vi "Tracker_v.2.2+.vi"() -> ()   [LabVIEW 2018]
uses:
  SubVi's/Controls/CTL_IO_parameters_indicator.ctl
  SubVi's/Controls/CTL_Zones_control_and_indicator.ctl
  SubVi's/Controls/CTL_All_References.ctl
  SubVi's/Controls/CTL_Controls_References.ctl
  SubVi's/Controls/CTL_Indicators_References.ctl
  SubVi's/Controls/CTL_Panes_and_VIs_References.ctl
  <vilib>/event_ctls.llb/eventsource.ctl
  SubVi's/Controls/CTL_Control_States.ctl
  <vilib>/Platform/TimedLoop/XDataNode/timing_clust.ctl
  <vilib>/Platform/TimedLoop/XDataNode/nitl_modes.ctl
  <vilib>/Platform/TimedLoop/XDataNode/wakeup.ctl
  <vilib>/Utility/error.llb/DialogType.ctl
  <vilib>/Instr/_visa.llb/VISA Flush IO Buffer Mask.ctl
  SubVi's/SW_Globals_2.2+.vi
  <vilib>/Platform/TimedLoop/scheduler/LVUserAPI/_suppVIs/Create_1kHz_TSource.vi
  <vilib>/platform/TimedLoop/XDataNode/XDataNode.xnode
  <vilib>/Platform/TimedLoop/XDataNode/XDNodeRunTimeDep.lvlib
panel:
  out "ItemPath":string
  out "ItemTag":string
  out "Source":T1 items=["LabVIEW UI"=0, "ActiveX"=1, "User Event"=25]
  out "Timing Source":string
  in  "Show magnets":bool=TRUE caption="Magnets"
  in  "Panes references":T2
  in  "Indicators references":T3
  in  "Controls references":T4
  in  "All references":T5
  out "Experiment Diagram":T6(plugin-control)
  in  "Reset barplot":bool
  out "Mouse speed, mm/s":dbl=0.28949046360238656 caption="Mouse speed" format="%05.1f"
  in  "Multiplyer of chart RX":u8(slide)=1 min=1 max=10 step=1 scale=1.0..6.0
  out "Running, perc. of time":dbl=0.28949046360238656 caption="Run, %" format="%05.2f"
  out "HW info":string
  out "Port":string="Large"
  in  "Reset stimuli":bool
  out "Ready":bool=TRUE
  in  "Check HW connection":bool
  in  "Reset zones":bool
  in  "Start Tracking button":bool
  in  "Playback speed":u16(ring)=3 caption="Speed" items=["25"=75, "10"=30, "6"=18, "4"=12, "2"=6, "1"=3, "2/3"=2, "1/3"=1]
  in  "Show heatmap":bool caption="Heat map"
  in  "Show full track":bool caption="Full track"
  in  "Timeline":dbl(slide) min=0.0 step=1.0 scale=0.0..3599.0 scale format="%<%H:%M:%S>t"
  in  "Play/Pause":bool
  in  "Open File":bool
  out "Record timestamp":dbl format="%<%H:%M:%S%3u>t"
  out "Current Time":timestamp=timestamp(3610093053.229 s since 1904-01-01) format="%<%H:%M:%S %d.%m.%Y>T"
  out "Current zone":T7={"01"=TRUE, "02"=TRUE, "03"=TRUE, "04"=TRUE, "05"=TRUE, "06"=TRUE, "07"=TRUE, "08"=TRUE, "09"=TRUE, "10"=TRUE, "11"=TRUE, "12"=TRUE, "13"=TRUE}
  in  "Show zones":bool=TRUE caption="Zones"
  in  "Trace, s":u16(slide)=5 max=30 step=1 scale=0.0..30.0
  in  "Record/Stop":bool
  out "Histograms":dbl[](graph) caption="Zone preference (normalized)"
  out "Mouse speed":waveform(dbl)(graph)={"t0"=timestamp(3610093053.229 s since 1904-01-01), "dt"=1.0, "Y"=[0.28949046360238656]}
  in  "By Zone stim. setup":T8=enum."Zone 13"
  out "IO status indicator":T9
  in  "error in (no error)":errorcluster
  out "error out":errorcluster={"status"=TRUE, "code"=1, "source"="Dequeue Element in NI_LVConfig.lvlib:Read Value Without Comment.vi->NI_LVConfig.lvlib:Read Key (I32).vi->SW_Load_settings_to_main_tab.vi"}
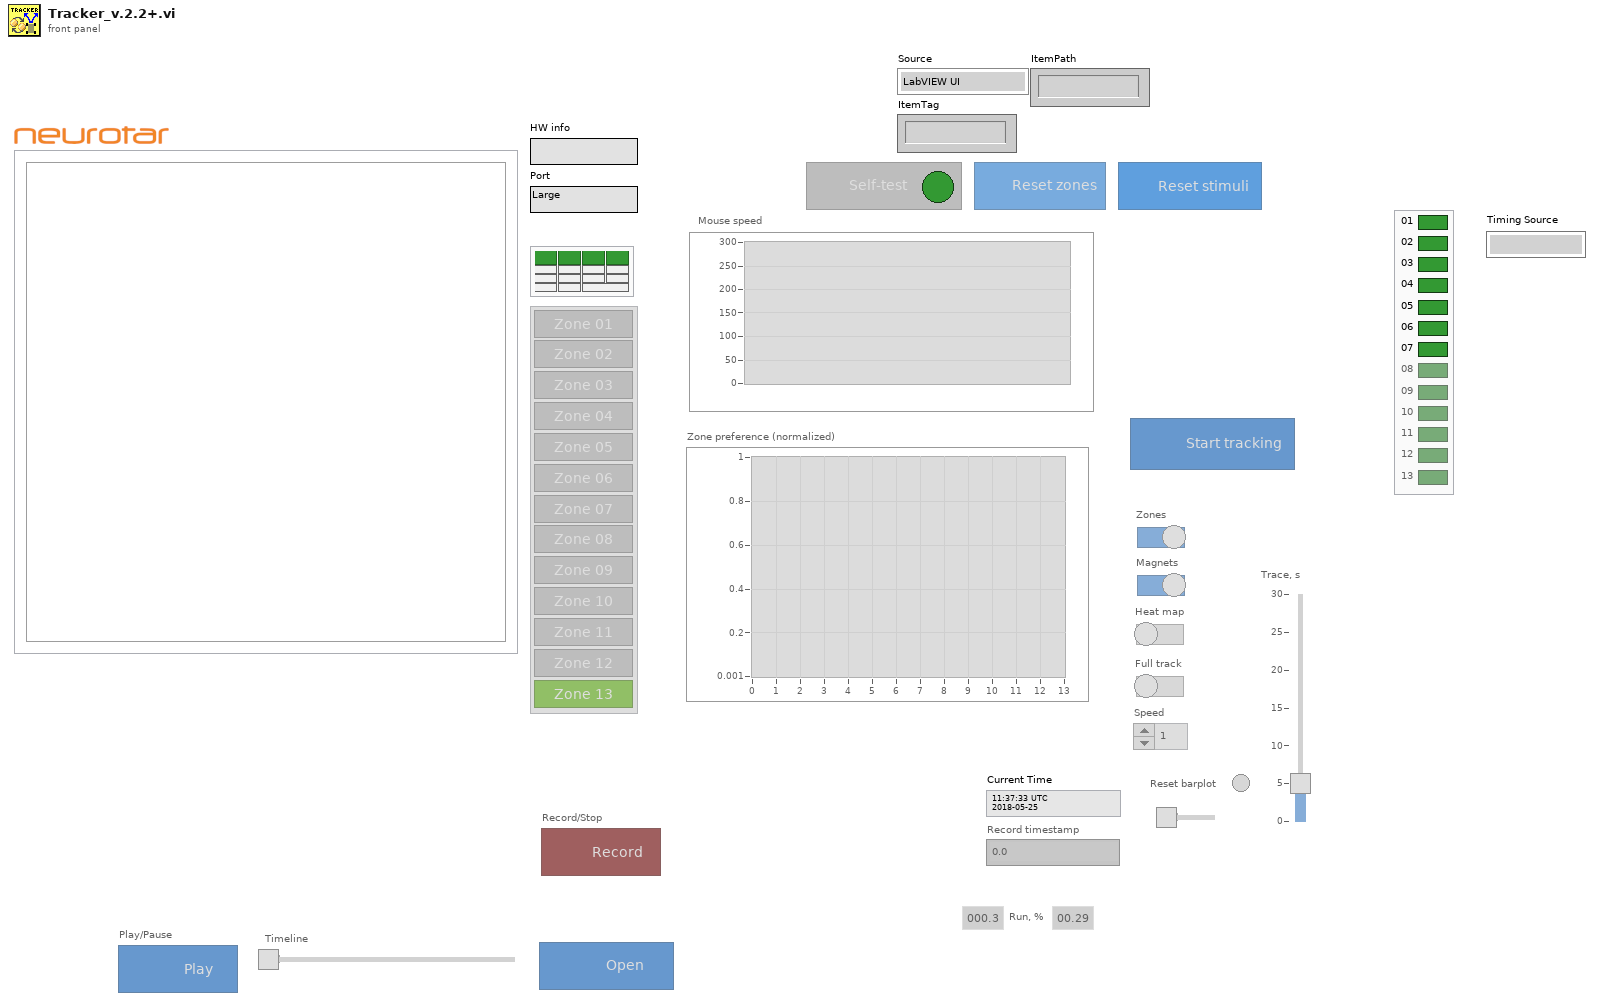
[diagram p1: front panel]
types:
  T1 = typedef "eventsource.ctl" = u32
  T2 = typedef "CTL_Panes_and_VIs_References.ctl" = cluster{"Pane":refnum<vi>, "This VI":refnum<vi>}
  T3 = typedef "CTL_Indicators_References.ctl" = cluster{"HW info":refnum<vi>, "Port":refnum<vi>, "Ready":refnum<vi>, "IO status indicator":refnum<vi>, "Current Time":refnum<vi>, "Record timestamp":refnum<vi>, "Mouse speed":refnum<vi>, "Mouse speed, mm/s":refnum<vi>, "Running, perc. of time":refnum<vi>, "Histograms":refnum<vi>}
  T4 = typedef "CTL_Controls_References.ctl" = cluster{"Check HW connection":refnum<vi>, "Start Tracking button":refnum<vi>, "Reset zones":refnum<vi>, "Reset stimuli":refnum<vi>, "Record/Stop":refnum<vi>, "Reset barplot":refnum<vi>, "Multiplyer of chart RX":refnum<vi>, "Show zones":refnum<vi>, "Show magnets":refnum<vi>, "Show heatmap":refnum<vi>, "Show full track":refnum<vi>, "Open File":refnum<vi>, "Play/Pause":refnum<vi>, "Trace, s":refnum<vi>, "Playback speed":refnum<vi>, "Timeline":refnum<vi>, "By Zone stim. setup":refnum<vi>}
  T5 = typedef "CTL_All_References.ctl" = cluster{"Controls references":T4, "Indicators references":T3, "Panes references":T2}
  T6 = typedef "IMAQ Image.ctl" = refnum<image>
  T7 = cluster{"01":bool, "02":bool, "03":bool, "04":bool, "05":bool, "06":bool, "07":bool, "08":bool, "09":bool, "10":bool, "11":bool, "12":bool, "13":bool}
  T8 = typedef "CTL_Zones_control_and_indicator.ctl" = enum32{"No Selection", "Zone 01", "Zone 02", "Zone 03", "Zone 04", "Zone 05", "Zone 06", "Zone 07", "Zone 08", "Zone 09", "Zone 10", "Zone 11", "Zone 12", "Zone 13"}
  T9 = typedef "CTL_IO_parameters_indicator.ctl" = cluster{"IO1":bool, "IO2":bool, "IO3":bool, "IO4":bool, "Z1":bool, "Z2":bool, "Z3":bool, "Z4":bool, "St1":bool, "St2":bool, "St3":bool, "St4":bool, "Syn1":bool, "Syn2":bool, "RS-232 ext. activated":bool}
  T10 = cluster{"HW info":refnum<vi>, "Port":refnum<vi>, "Ready":refnum<vi>, "IO status indicator":refnum<vi>, "Current Time":refnum<vi>, "Record timestamp":refnum<vi>, "Mouse speed":refnum<vi>, "Mouse speed, mm/s":refnum<vi>, "Running, perc. of time":refnum<vi>, "Histograms":refnum<vi>}
  T11 = cluster{"Check HW connection":refnum<vi>, "Start Tracking button":refnum<vi>, "Reset zones":refnum<vi>, "Reset stimuli":refnum<vi>, "Record/Stop":refnum<vi>, "Reset barplot":refnum<vi>, "Multiplyer of chart RX":refnum<vi>, "Show zones":refnum<vi>, "Show magnets":refnum<vi>, "Show heatmap":refnum<vi>, "Show full track":refnum<vi>, "Open File":refnum<vi>, "Play/Pause":refnum<vi>, "Trace, s":refnum<vi>, "Playback speed":refnum<vi>, "Timeline":refnum<vi>, "By Zone stim. setup":refnum<vi>}
  T12 = typedef "CTL_Control_States.ctl" = enum16{"SW Init", "HW Init", "Close App"}
  T13 = typedef "XDNodeRunTimeDep.lvlib/timing_clust.ctl" = cluster{"Expected End [f-1]":u64, "Actual End [f-1]":u64, "Finished Late? [f-1]":bool, "Expected End [i-1]":u64, "Actual End [i-1]":u64, "Finished Late? [i-1]":bool, "Expected Start [i]":u64, "Actual Start [i]":u64, "Expected Start [f]":u64, "Actual Start [f]":u64, "Source Name":string, "Structure Name":string, "Period":i64, "Deadline":i64, "Offset":i64, "Start":i64, "Priority":i32, "Timeout":i32, "Mode":T14, "Wakeup Reason":T15, "Error":errorcluster, "Source Type":string, "Secondary Source Type":string, "Global End Time":u64, "Global Start Time":u64, "Frame Duration":u64, "Iteration Duration":u64, "Assigned CPU":i32, "I/O Scan Engine Mode":u32}
  T14 = typedef "XDNodeRunTimeDep.lvlib/nitl_modes.ctl" = enum32{"No Change", "Process missed periods, maintain original phase", "Discard missed periods, maintain original phase", "Process missed periods, ignore original phase", "Discard missed periods, ignore original phase"}
  T15 = typedef "XDNodeRunTimeDep.lvlib/wakeup.ctl" = enum32{"Normal", "Aborted", "Asynchronous wakeup", "Timing source error", "Timed loop error", "Timeout"}
  T16 = typedef "DialogType.ctl" = u16
  T17 = enum32{"invalid app kind", "Development System", "Run Time System", "Student Edition", "Embedded LabVIEW", "Evaluation", "Custom"}
  T18 = typedef "CTL_Settings_cluster.ctl" = cluster{"Defaults":cluster{"Default User":dbl, "VISA Resource Name ":string}, "Recording and saving":cluster{"Researcher name":string, "Name prefix":string, "Data filtering":u16, "Stop at":dbl, "\"Stop at\" enabled":bool}, "Geometry":cluster{"Cage diameter, mm":u16, "Starting angle MIDFIELD":i16, "Starting angle BORDER":i16, "Radius, mm CENTER":u16, "Radius, mm MIDFIELD":u16, "N segments MIDFIELD":u8, "N segments BORDER":u8, "R-gap, mm":sgl, "Bridge swap":bool, "Bridge H. offset":sgl, "Bridge V. offset":sgl, "Twisted neck":bool}, "IO parameters":cluster{"SYNC configuration":u16, "IO 1 configuration":u16, "IO 2 configuration":u16, "IO 3 configuration":u16, "IO 4 configuration":u16, "Activate ext. RS-232":u16, "IO inversion config.":u16}, "Stimulus presets array":T19[], "Settings loaded OK":bool}
  T19 = typedef "CTL_Single_stimulus_setting.ctl" = cluster{"Event type":u16, "Dur., s":sgl, "Stim., s":sgl, "TTL out N":u16, "Set/Clear":bool, "Stim. has been set":bool}
  T20 = typedef "CTL_Paths_cluster.ctl" = cluster{"Temporary file output path":path, "Density map array output path":path, "Recording settings output path":path, "Density map picture output path":path, "Layout picture output path":path, "Path to the settings file":path, "Path to TDMS file":path, "TDMS file reference":refnum<k34>}
  T21 = typedef "VISA Flush IO Buffer Mask.ctl" = u16
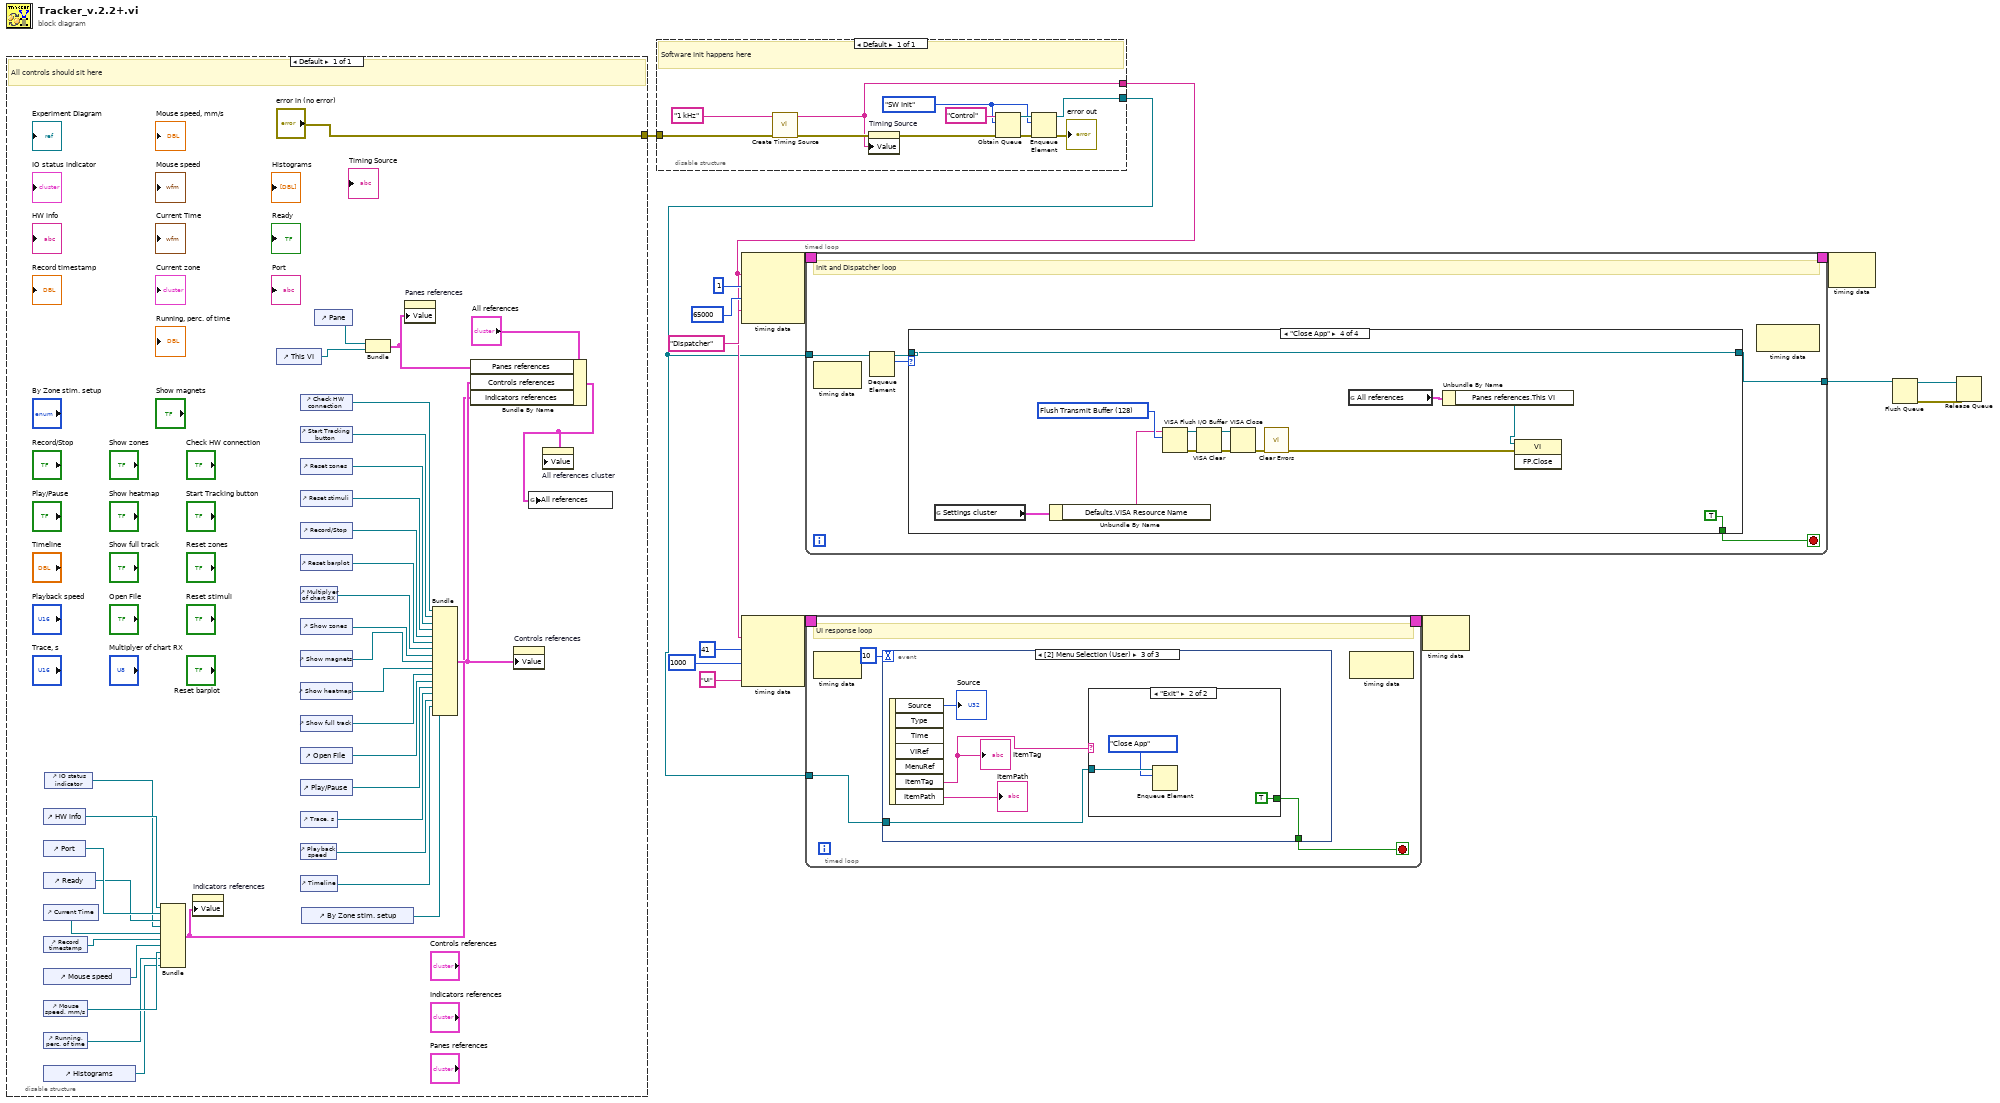
[diagram p0: block diagram]
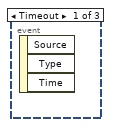
[diagram p2: hidden frame]
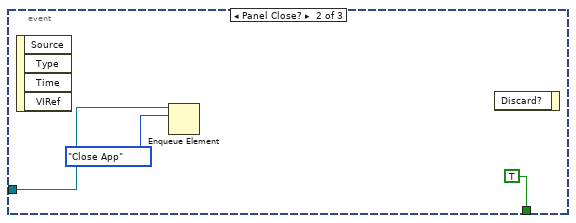
[diagram p3: hidden frame]
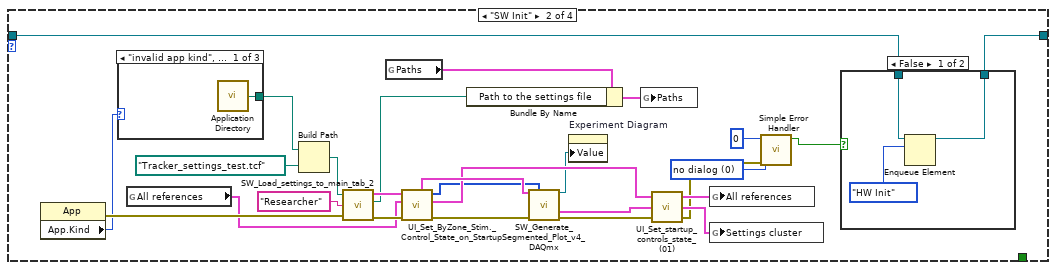
[diagram p6: hidden frame]
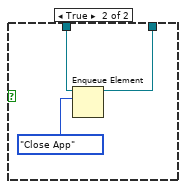
[diagram p7: hidden frame]
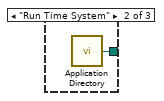
[diagram p8: hidden frame]
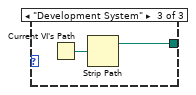
[diagram p9: hidden frame]
diagram:
  n1 = disable-structure shown="Default" {
    disable-tunnel: ["error in (no error)"] -> w11
    frame Enabled {
      # "All controls should sit here"
      n2 = control-ref of="HW info"() -> (w34:refnum<vi>)
      n3 = control-ref of="Port"() -> (w33:refnum<vi>)
      n4 = control-ref of="Ready"() -> (w32:refnum<vi>)
      n5 = control-ref of="Current Time"() -> (w31:refnum<vi>)
      n6 = control-ref of="Record timestamp"() -> (w30:refnum<vi>)
      n7 = control-ref of="Mouse speed"() -> (w29:refnum<vi>)
      n8 = control-ref of="Mouse speed, mm/s"() -> (w28:refnum<vi>)
      n9 = control-ref of="Running, perc. of time"() -> (w27:refnum<vi>)
      n10 = control-ref of="Histograms"() -> (w26:refnum<vi>)
      n11 = control-ref of="IO status indicator"() -> (w22:refnum<vi>)
      n12 = Bundle("HW info"=w34, "Port"=w33, "Ready"=w32, "IO status indicator"=w22, "Current Time"=w31, "Record timestamp"=w30, "Mouse speed"=w29, "Mouse speed, mm/s"=w28, "Running, perc. of time"=w27, "Histograms"=w26) -> (w18:T10)  [unwired: 1 in]
      n13 = property on="Indicators references" class="Clust (strict)"("Value"=w18) -> ()  [unwired: 2 in, 2 out]
      n14 = control-ref of="This VI"() -> (w24:refnum<vi>)
      n15 = control-ref of="Check HW connection"() -> (w50:refnum<vi>)
      n16 = control-ref of="Start Tracking button"() -> (w49:refnum<vi>)
      n17 = control-ref of="Reset zones"() -> (w48:refnum<vi>)
      n18 = control-ref of="Reset stimuli"() -> (w47:refnum<vi>)
      n19 = control-ref of="Record/Stop"() -> (w46:refnum<vi>)
      n20 = control-ref of="Reset barplot"() -> (w45:refnum<vi>)
      n21 = control-ref of="Multiplyer of chart RX"() -> (w44:refnum<vi>)
      n22 = control-ref of="Show zones"() -> (w43:refnum<vi>)
      n23 = control-ref of="Show magnets"() -> (w23:refnum<vi>)
      n24 = control-ref of="Show heatmap"() -> (w42:refnum<vi>)
      n25 = control-ref of="Show full track"() -> (w41:refnum<vi>)
      n26 = control-ref of="Open File"() -> (w40:refnum<vi>)
      n27 = control-ref of="Play/Pause"() -> (w39:refnum<vi>)
      n28 = control-ref of="Trace, s"() -> (w38:refnum<vi>)
      n29 = control-ref of="Playback speed"() -> (w37:refnum<vi>)
      n30 = control-ref of="Timeline"() -> (w36:refnum<vi>)
      n31 = control-ref of="By Zone stim. setup"() -> (w35:refnum<vi>)
      n32 = control-ref of="Pane"() -> (w25:refnum<vi>)
      n33 = Bundle("Pane"=w25, "This VI"=w24) -> (w20:cluster{"Pane":refnum<vi>, "This VI":refnum<vi>})  [unwired: 1 in]
      n34 = property on="Panes references" class="Clust (strict)"("Value"=w20) -> ()  [unwired: 2 in, 2 out]
      n35 = Bundle("Check HW connection"=w50, "Start Tracking button"=w49, "Reset zones"=w48, "Reset stimuli"=w47, "Record/Stop"=w46, "Reset barplot"=w45, "Multiplyer of chart RX"=w44, "Show zones"=w43, "Show magnets"=w23, "Show heatmap"=w42, "Show full track"=w41, "Open File"=w40, "Play/Pause"=w39, "Trace, s"=w38, "Playback speed"=w37, "Timeline"=w36, "By Zone stim. setup"=w35) -> (w19:T11)  [unwired: 1 in]
      n36 = Bundle By Name(cluster="All references", "Panes references"=w20, "Controls references"=w19, "Indicators references"=w18) -> (w17:T5)
      n37 = property on="Controls references" class="Clust (strict)"("Value"=w19) -> ()  [unwired: 2 in, 2 out]
      n38 = global write "SW_Globals_2.2+.vi" "All references"(w17) -> ()
      n39 = property on="All references cluster" class="Clust (strict)"("Value"=w17) -> ()  [unwired: 2 in, 2 out]
    }
  }
  n40 = disable-structure shown="Default" {
    disable-tunnel: [w61] -> w5
    disable-tunnel: [w53] -> w1
    disable-tunnel: w11 -> [w52]
    frame Enabled {
      w54 = CTL_Control_States."SW Init"
      # "Software Init happens here"
      n41 = call-poly <vilib>:"Create Timing Source.vi"("error in (no error)"=w52, "name (in)"="1 kHz") -> ("error out"=w62:errorcluster, "name (out)"=w61:string)  [unwired: 8 in]
      n42 = property on="Timing Source" class="Str"(error in=w62, "Value"=w61) -> (error out=w59:errorcluster)  [unwired: 1 in, 1 out]
      n43 = Obtain Queue(name (unnamed)="Control", element data type=w54, error in (no error)=w59) -> (queue out=w56:refnum<queue>, error out=w57:errorcluster)  [unwired: 2 in, 1 out]
      n44 = Enqueue Element(queue=w56, element=w54, error in (no error)=w57) -> (queue out=w53:refnum<queue>, error out=→"error out":errorcluster)  [unwired: 1 in, 1 out]
    }
  }
  n45 = node-c288(w5, i64 1 ("Period"), 65000 ("Priority"), "Dispatcher" ("Structure Name")) -> (w16:T13)
  n46 = node-c288(w5, i64 41 ("Period"), 1000 ("Priority"), "UI" ("Structure Name")) -> (w7:T13)
  n47 = timed-loop {
    timing: w16 -> [_]
    timing-out: [_] -> w15
    tunnel: w1 -> [w67]
    tunnel: [w64] -> w9
    stop <- w63 stop-if-true
    # "Init and Dispatcher loop"
    n48 = node-c288() -> ()  [unwired: 1 in, 1 out]
    n49 = Dequeue Element(queue=w67) -> (queue out=w65:refnum<queue>, element=w66:T12)  [unwired: 2 in, 2 out]
    n50 = case shown="\"Close App\"" w66 {
      tunnel: [w68 w70 w106 w119] -> w64
      tunnel: w65 -> [w68 w71 w106 w119]
      tunnel: [_ _ _ TRUE] -> w63
      frame Default {
      }
      frame "SW Init" {
        w73 = T16 0 items=["no dialog", "OK message", "continue or stop message", "OK message + warnings", "continue/stop + warnings"] ("type of dialog (OK msg:1)")
        n51 = property class="App"() -> (error out=w83:errorcluster, "App.Kind"=w77:T17)  [unwired: 2 in, 1 out]
        n52 = case shown="\"invalid app kind\", Default" w77 {
          tunnel: [w102 w103 w104] -> w78
          frame "invalid app kind", Default {
            n53 = call <vilib>:"Application Directory.vi"() -> ("Application Directory"=w102:path)
          }
          frame "Run Time System" {
            n54 = call <vilib>:"Application Directory.vi"() -> ("Application Directory"=w103:path)
          }
          frame "Development System" {
            n55 = Current VI's Path() -> (path=w105:path)
            n56 = Strip Path(path=w105) -> (stripped path=w104:path)  [unwired: 1 out]
          }
        }
        n57 = global read "SW_Globals_2.2+.vi" "All references"() -> (w69:T5)
        n58 = Build Path(base path=w78, name or relative path=path "Tracker_settings_test.tcf") -> (appended path=w95:path)
        n59 = call "SW_Load_settings_to_main_tab_2.vi"("Settings path in"=w95, "Researcher name"="Researcher", "error in (no error)"=w83) -> ("Settings cluster out"=w87:T18, "Settings file path"=w80:path, "error out"=w92:errorcluster)  [unwired: 5 in]
        n60 = global read "SW_Globals_2.2+.vi" "Paths"() -> (w82:T20)
        n61 = call "UI_Set_ByZone_Stim._Control_State_on_Startup.vi"("Error In"=w92, "All references cluster"=w69, "Settings cluster"=w87) -> ("Error Out"=w89:errorcluster, "All references cluster out"=w86:T5, "Regions to track"=w85:u8[], "Settings cluster out"=w88:T18)  [unwired: 5 in]
        n62 = Bundle By Name(cluster=w82, "Path to the settings file"=w80) -> (w81:T20)
        n63 = call "SW_Generate_Segmented_Plot_v4_DAQmx.vi"("Settings cluster in"=w88, "Regions to mark set (none)"=w85, "Error In"=w89) -> ("Experiment Diagram"=w84:T6, "Settings cluster out"=w91:T18, "Error Out"=w90:errorcluster)  [unwired: 8 in, 2 out]
        n64 = property on="Experiment Diagram" class="ImageControl"("Value"=w84) -> ()  [unwired: 2 in, 2 out]
        n65 = global write "SW_Globals_2.2+.vi" "Paths"(w81) -> ()
        n66 = call "UI_Set_startup_controls_state_(01).vi"("error in (no error)"=w90, "Settings cluster in"=w91, "All references in"=w86) -> ("error out"=w75:errorcluster, "Settings cluster out"=w93:T18, "All references out"=w94:T5)
        n67 = global write "SW_Globals_2.2+.vi" "All references"(w94) -> ()
        n68 = global write "SW_Globals_2.2+.vi" "Settings cluster"(w93) -> ()
        n69 = call <vilib>:"Simple Error Handler.vi"("error code (no error:0)"=0, "type of dialog (OK msg:1)"=w73, "error in (no error)"=w75) -> ("error?"=w72:bool)  [unwired: 2 in, 4 out]
        n70 = case shown="False" w72 {
          tunnel: w71 -> [w98 w101]
          tunnel: [w97 w100] -> w70
          frame False {
            n71 = Enqueue Element(queue=w98, element=CTL_Control_States."HW Init") -> (queue out=w97:refnum<queue>)  [unwired: 2 in, 2 out]
          }
          frame True {
            n72 = Enqueue Element(queue=w101, element=CTL_Control_States."Close App") -> (queue out=w100:refnum<queue>)  [unwired: 2 in, 2 out]
          }
        }
      }
      frame "HW Init" {
      }
      frame "Close App" {
        w113 = T21 128 items=["Flush Receive Buffer"=16, "Write Transmit Buffer to Device"=32, "Flush Receive Buffer (No I/O)"=64, "Flush Transmit Buffer"=128] ("Mask")
        n73 = global read "SW_Globals_2.2+.vi" "Settings cluster"() -> (w112:T18)
        n74 = Unbundle By Name(w112) -> ("Defaults.VISA Resource Name"=w111:string)
        n75 = VISA Flush I/O Buffer(VISA resource name=w111, mask (16)=w113) -> (VISA resource name out=w114:refnum<visa-resource-name>, error out=w115:errorcluster)  [unwired: 1 in]
        n76 = VISA Clear(VISA resource name=w114, error in (no error)=w115) -> (VISA resource name out=w117:refnum<visa-resource-name>, error out=w116:errorcluster)
        n77 = VISA Close(VISA resource name=w117, error in (no error)=w116) -> (error out=w118:errorcluster)
        n78 = call <vilib>:"Clear Errors.vi"("error in (no error)"=w118) -> ("error out"=w109:errorcluster)  [unwired: 5 in, 1 out]
        n79 = global read "SW_Globals_2.2+.vi" "All references"() -> (w110:T5)
        n80 = Unbundle By Name(w110) -> ("Panes references.This VI"=w108:refnum<vi>)
        n81 = invoke class="VI" method="FP.Close"(reference=w108, error in=w109) -> ()  [unwired: 1 in, 3 out]
      }
    }
    n82 = node-c288() -> ()  [unwired: 1 in, 1 out]
  }
  n83 = timed-loop {
    timing: w7 -> [_]
    timing-out: [_] -> w6
    tunnel: w1 -> [w123]
    stop <- w124 stop-if-true
    # "UI response loop"
    n84 = node-c288() -> ()  [unwired: 1 in, 1 out]
    n85 = event shown="[2] Menu Selection (User)" {
      selector: _ -> [_ _ _]
      dyn-events: _ -> [_ _ _]
      timeout: 10 -> [_ _ _]
      tunnel: [_ TRUE w128] -> w124
      tunnel: w123 -> [_ w126 w129]
      event Timeout {
        n86 = event-data() -> ()  [unwired: 1 in, 3 out]
      }
      event Panel Close? {
        n87 = event-data() -> ()  [unwired: 1 in, 4 out]
        n88 = Enqueue Element(queue=w126, element=CTL_Control_States."Close App") -> ()  [unwired: 2 in, 3 out]
        n89 = event-data() -> ()  [unwired: 2 in, 1 out]
      }
      event Menu Selection (User) {
        n90 = event-data() -> ("Source"=→"Source":T1, "ItemTag"=w130:string, "ItemPath"=→"ItemPath":string)  [unwired: 1 in, 4 out]
        "ItemTag" <- w130
        n91 = case shown="\"Exit\"" w130 {
          tunnel: w129 -> [_ w135]
          tunnel: [_ TRUE] -> w128
          frame "\u0000", Default {
          }
          frame "Exit" {
            n92 = Enqueue Element(queue=w135, element=CTL_Control_States."Close App") -> ()  [unwired: 2 in, 3 out]
          }
        }
      }
    }
    n93 = node-c288() -> ()  [unwired: 1 in, 1 out]
  }
  n94 = node-c288(w6) -> ()  [unwired: 1 out]
  n95 = node-c288(w15) -> ()  [unwired: 1 out]
  n96 = Flush Queue(queue=w9) -> (queue out=w8:refnum<queue>, error out=w10:errorcluster)  [unwired: 1 in, 1 out]
  n97 = Release Queue(queue=w8, error in (no error)=w10) -> ()  [unwired: 1 in, 3 out]
